vi "MergeTwoWaves.vi"() -> ()   [LabVIEW 2019]
panel:
  in  "Stop Merging":bool
  out "Waveform Chart":dynamicdata(graph)
  in  "Amplitude":dbl(knob) scale=0.0..100.0
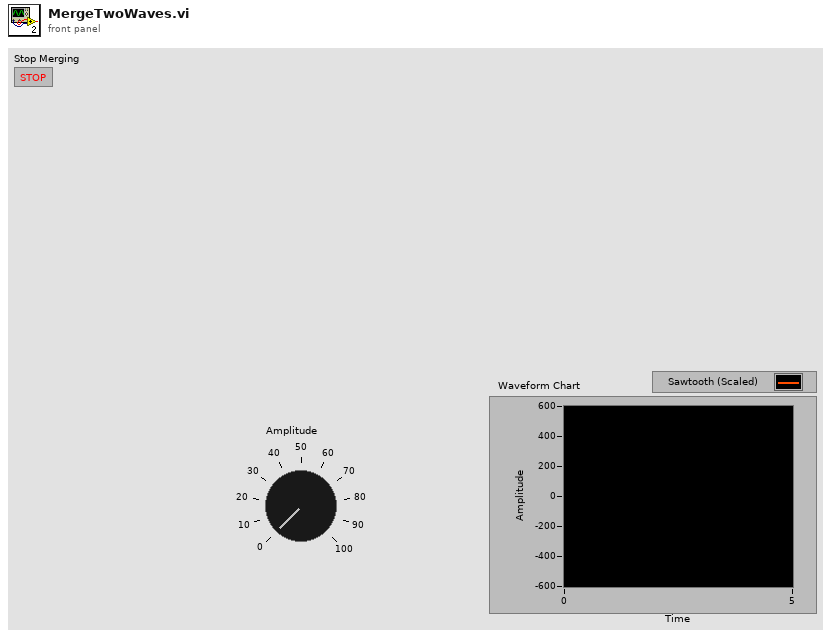
[diagram p1: front panel]
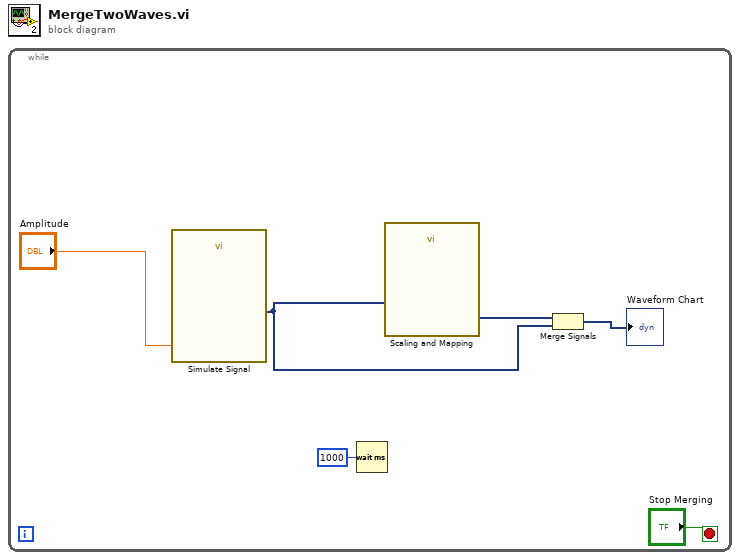
[diagram p0: block diagram]
diagram:
  n1 = while {
    stop <- "Stop Merging" stop-if-true
    n2 = call "Simulate Signal"("Amplitude"="Amplitude") -> ("Sawtooth"=w5:dynamicdata)  [unwired: 13 in, 1 out]
    n3 = Wait (ms)(milliseconds to wait=u32 1000) -> ()  [unwired: 1 out]
    n4 = call "Scaling and Mapping"("Signals"=w5) -> ("Scaled Signals"=w4:dynamicdata)  [unwired: 9 in, 1 out]
    n5 = Merge Signals "Merge Signals"(w4, w5) -> (→"Waveform Chart":dynamicdata)
  }
